vi "visiontest.vi"(0 "Image Src":T1, 7 "error in":errorcluster) -> (20 "Number of Particles (Particle Analysis 1)":i32, 21 "Particle Measurements (Pixels) (Particle Analysis 1)":dbl[][](array[numeric]) format="%.2f", 27 "error out":errorcluster)   [LabVIEW 2011]
uses:
  <vilib>/vision/Image Controls.llb/IMAQ Image.ctl
  <vilib>/vision/NI_Vision_Development_Module.lvlib
panel:
  out "Image Out":T1(plugin-control)
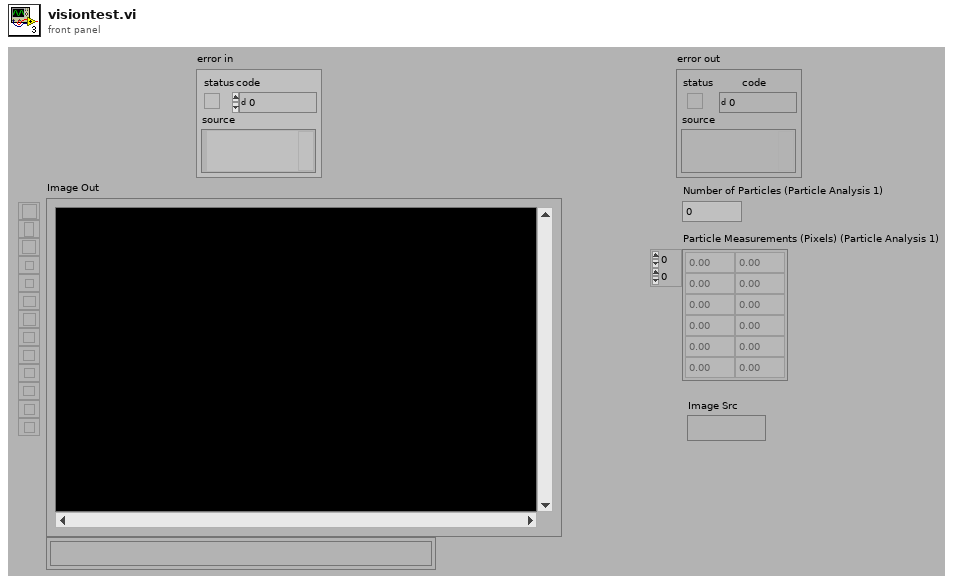
[diagram p1: front panel]
types:
  T1 = typedef "IMAQ Image.ctl" = refnum<image>
  T2 = cluster{"Measurement Parameter":i32, "Range Lower Value":dbl, "Range Upper Value":dbl, "Range":bool, "Measurement Type":bool}[]
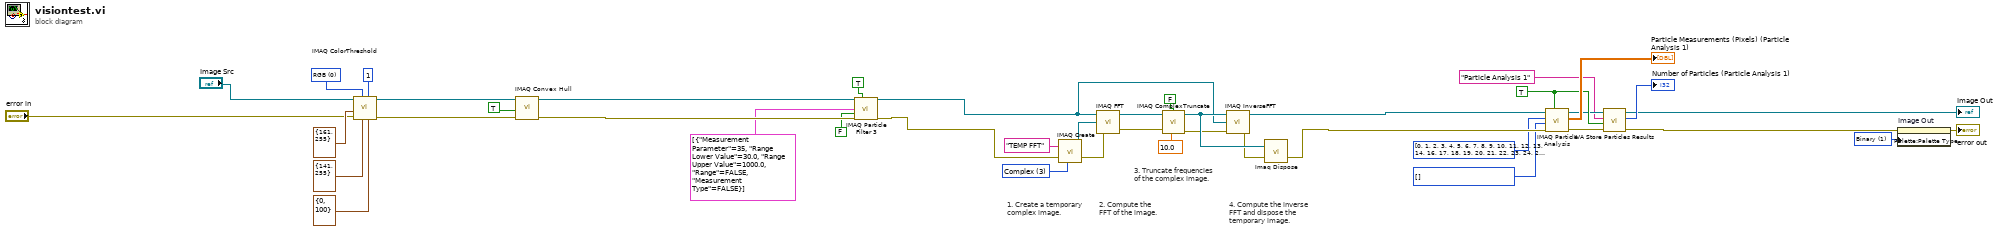
[diagram p0: block diagram]
diagram:
  w4 = u32 1 items=["Grayscale", "Binary", "Gradient", "Rainbow", "Temperature", "User Defined"] ("Palette")
  w14 = i32[] [] items=["Center of Mass X", "Center of Mass Y", "First Pixel X", "First Pixel Y", "Bounding Rect Left", "Bounding Rect Top", "Bounding Rect Right", "Bounding Rect Bottom", "Max Feret Diameter Start X", "Max Feret Diameter Start Y", "Max Feret Diameter End X", "Max Feret Diameter End Y", "Max Horiz. Segment Length Left", "Max Horiz. Segment Length Right", "Max Horiz. Segment Length Row", "-", "Bounding Rect Width", "Bounding Rect Height", "Bounding Rect Diagonal", "Perimeter", "Convex Hull Perimeter", "Holes' Perimeter", "Max Feret Diameter", "Equivalent Ellipse Major Axis", "Equivalent Ellipse Minor Axis", "Equivalent Ellipse Minor Axis (Feret)", "Equivalent Rect Long Side", "Equivalent Rect Short Side", "Equivalent Rect Diagonal", "Equivalent Rect Short Side (Feret)", "Average Horiz. Segment Length", "Average Vert. Segment Length", "Hydraulic Radius", "Waddel Disk Diameter", "-", "Area", "Holes' Area", "Particle & Holes' Area", "Convex Hull Area", "Image Area", "-", "Number of Holes", "Number of Horiz. Segments", "Number of Vert. Segments", "-", "Orientation", "Max Feret Diameter Orientation", "-", "% Area/Image Area", "% Area/(Particle & Holes' Area)", "Ratio of Equivalent Ellipse Axes", "Ratio of Equivalent Rect Sides", "-", "Elongation Factor", "Compactness Factor", "Heywood Circularity Factor", "Type Factor", "-", "Sum X", "Sum Y", "Sum XX", "Sum XY", "Sum YY", "Sum XXX", "Sum XXY", "Sum XYY", "Sum YYY", "-", "Moment of Inertia XX", "Moment of Inertia XY", "Moment of Inertia YY", "Moment of Inertia XXX", "Moment of Inertia XXY", "Moment of Inertia XYY", "Moment of Inertia YYY", "Norm. Moment of Inertia XX", "Norm. Moment of Inertia XY", "Norm. Moment of Inertia YY", "Norm. Moment of Inertia XXX", "Norm. Moment of Inertia XXY", "Norm. Moment of Inertia XYY", "Norm. Moment of Inertia YYY", "Hu Moment 1", "Hu Moment 2", "Hu Moment 3", "Hu Moment 4", "Hu Moment 5", "Hu Moment 6", "Hu Moment 7"] ("Real-World Measurements")
  w15 = i32[] [0, 1, 2, 3, 4, 5, 6, 7, 8, 9, 10, 11, 12, 13, 14, 16, 17, 18, 19, 20, 21, 22, 23, 24, 25, 26, 27, 28, 29, 30, 31, 32, 33, 35, 36, 37, 38, 39, 41, 42, 43, 45, 46, 48, 49, 50, 51, 53, 54, 55, 56, 58, 59, 60, 61, 62, 63, 64, 65, 66, 68, 69, 70, 71, 72, 73, 74, 75, 76, 77, 78, 79, 80, 81, 82, 83, 84, 85, 86, 87, 88] items=["Center of Mass X", "Center of Mass Y", "First Pixel X", "First Pixel Y", "Bounding Rect Left", "Bounding Rect Top", "Bounding Rect Right", "Bounding Rect Bottom", "Max Feret Diameter Start X", "Max Feret Diameter Start Y", "Max Feret Diameter End X", "Max Feret Diameter End Y", "Max Horiz. Segment Length Left", "Max Horiz. Segment Length Right", "Max Horiz. Segment Length Row", "-", "Bounding Rect Width", "Bounding Rect Height", "Bounding Rect Diagonal", "Perimeter", "Convex Hull Perimeter", "Holes' Perimeter", "Max Feret Diameter", "Equivalent Ellipse Major Axis", "Equivalent Ellipse Minor Axis", "Equivalent Ellipse Minor Axis (Feret)", "Equivalent Rect Long Side", "Equivalent Rect Short Side", "Equivalent Rect Diagonal", "Equivalent Rect Short Side (Feret)", "Average Horiz. Segment Length", "Average Vert. Segment Length", "Hydraulic Radius", "Waddel Disk Diameter", "-", "Area", "Holes' Area", "Particle & Holes' Area", "Convex Hull Area", "Image Area", "-", "Number of Holes", "Number of Horiz. Segments", "Number of Vert. Segments", "-", "Orientation", "Max Feret Diameter Orientation", "-", "% Area/Image Area", "% Area/(Particle & Holes' Area)", "Ratio of Equivalent Ellipse Axes", "Ratio of Equivalent Rect Sides", "-", "Elongation Factor", "Compactness Factor", "Heywood Circularity Factor", "Type Factor", "-", "Sum X", "Sum Y", "Sum XX", "Sum XY", "Sum YY", "Sum XXX", "Sum XXY", "Sum XYY", "Sum YYY", "-", "Moment of Inertia XX", "Moment of Inertia XY", "Moment of Inertia YY", "Moment of Inertia XXX", "Moment of Inertia XXY", "Moment of Inertia XYY", "Moment of Inertia YYY", "Norm. Moment of Inertia XX", "Norm. Moment of Inertia XY", "Norm. Moment of Inertia YY", "Norm. Moment of Inertia XXX", "Norm. Moment of Inertia XXY", "Norm. Moment of Inertia XYY", "Norm. Moment of Inertia YYY", "Hu Moment 1", "Hu Moment 2", "Hu Moment 3", "Hu Moment 4", "Hu Moment 5", "Hu Moment 6", "Hu Moment 7"] ("Pixel Measurements")
  w11 = TRUE ("Connectivity 4/8 (8)")
  w28 = u32 3 items=["8 bits", "16 bits", "Float", "Complex", "RGB", "HSL"] ("Image Type")
  w41 = u16 0 items=["RGB", "HSL", "HSV", "HSI"] ("Color Mode")
  # "4. Compute the inverse\nFFT and dispose the\ntemporary image."
  # "3. Truncate frequencies\nof the complex image."
  # "2. Compute the\nFFT of the image."
  # "1. Create a temporary\ncomplex image."
  n1 = call "IMAQ ColorThreshold"("Blue or Luma or Val or Inten Range"=cluster{"Lower value":i32, "Upper value":i32} {"Lower value"=0, "Upper value"=100}, "Replace Value"=1, "Green or Sat Range"=cluster{"Lower value":i32, "Upper value":i32} {"Lower value"=141, "Upper value"=255}, "Color Mode"=w41, "error in (no error)"="error in", "Red or Hue Range"=cluster{"Lower value":i32, "Upper value":i32} {"Lower value"=161, "Upper value"=255}, "Image Src"="Image Src") -> ("error out"=w37:errorcluster, "Image Dst Out"=w36:T1)  [unwired: 1 in, 2 out]
  n2 = call "IMAQ Convex Hull"("error in (no error)"=w37, "Connectivity 4/8 (8)"=TRUE, "Image Src"=w36) -> ("error out"=w34:errorcluster, "Image Dst Out"=w30:T1)  [unwired: 1 in, 6 out]
  n3 = call "IMAQ Particle Filter 3"("Image Src"=w30, "Connectivity 4/8 (8)"=TRUE, "Selection Values"=T2 [{"Measurement Parameter"=35, "Range Lower Value"=30.0, "Range Upper Value"=1000.0, "Range"=FALSE, "Measurement Type"=FALSE}], "Keep/Remove Particles (F)"=FALSE ("Keep/Remove Particles"), "error in (no error)"=w34) -> ("Image Dst Out"=w18:T1, "error out"=w31:errorcluster)  [unwired: 4 in, 5 out]
  n4 = call "IMAQ Create"("Image Name"="TEMP FFT", "Image Type"=w28, "error in (no error)"=w31) -> ("New Image"=w26:T1, "error out"=w19:errorcluster)  [unwired: 1 in, 1 out]
  n5 = call "IMAQ FFT"("error in (no error)"=w19, "Image Dst"=w26, "Image Src"=w18) -> ("error out"=w24:errorcluster, "Image Dst Out"=w25:T1)  [unwired: 1 out]
  n6 = call "IMAQ ComplexTruncate"("error in (no error)"=w24, "Truncation Frequency %"=sgl 10.0, "Image Src"=w25, "Low pass/High pass (Low pass)"=FALSE) -> ("error out"=w22:errorcluster, "Image Dst Out"=w23:T1)  [unwired: 1 in, 2 out]
  n7 = call "IMAQ InverseFFT"("error in (no error)"=w22, "Image Dst"=w18, "Image Src"=w23) -> ("error out"=w21:errorcluster, "Image Dst Out"=w12:T1)  [unwired: 1 out]
  n8 = call "Imaq Dispose"("Image"=w23, "error in (no error)"=w21) -> ("error out"=w20:errorcluster)  [unwired: 1 in, 3 out]
  n9 = call "IMAQ Particle Analysis"("Connectivity 4/8 (8)"=w11, "error in (no error)"=w20, "Real-World Measurements"=w14, "Pixel Measurements"=w15, "Image"=w12) -> ("error out"=w8:errorcluster, "Particle Measurements (Pixels)"=→"Particle Measurements (Pixels) (Particle Analysis 1)":dbl[][], "Image Out (duplicate)"=w10:T1)  [unwired: 4 out]
  n10 = call <vilib>:"IVA Store Particles Results.vi"("error in (no error)"=w8, "Connectivity 4/8 (8)"=w11, "Step Name"="Particle Analysis 1", "Image in"=w10) -> ("error out"=w7:errorcluster, "Number of Particles"=→"Number of Particles (Particle Analysis 1)":i32, "Image dup"=→"Image Out":T1)  [unwired: 5 out]
  n11 = property on="Image Out" class="ImageControl"(error in=w7, "Palette:Palette Type"=w4) -> (error out=→"error out":errorcluster)  [unwired: 1 in, 1 out]
